vi "String-Matrix.vi"(10 "String":string) -> (0 "error out":errorcluster, 2 "String Out":string, 3 "T":T1=[[0.016284994521607307, 0.9998576764567041, 0.0044074691186384496, -12.095922523672678], [0.9998670931969393, -0.01628143110047913, -0.0008431744914288715, -1019.3924117975101], [-0.0007712945830650122, 0.004420614427981981, -0.999989931585686, 240.25900755427352], [0.0, 0.0, 0.0, 1.0]] format="%.3f")   [LabVIEW 2013]
uses:
  <vilib>/Analysis/Matrix/Datatypes/RealMatrix.ctl
  <vilib>/Analysis/Matrix/NI_Matrix.lvlib
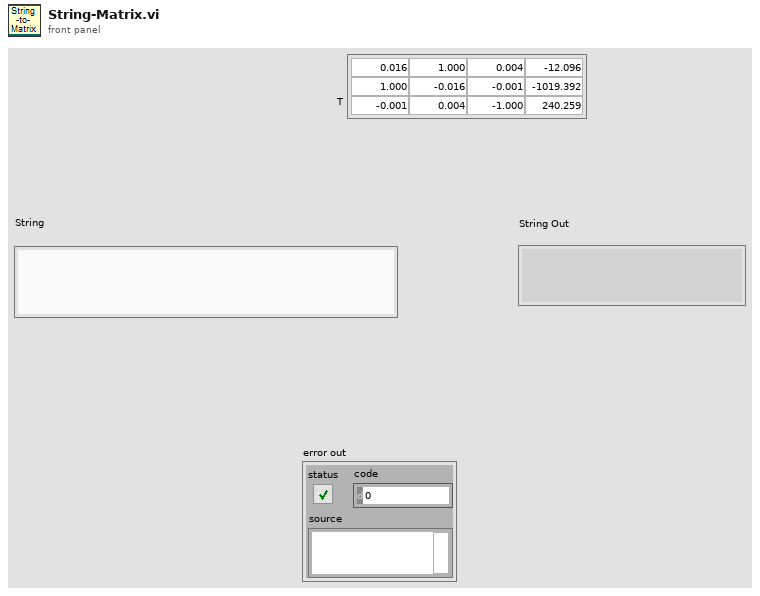
[diagram p1: front panel]
types:
  T1 = typedef "NI_Matrix.lvlib/RealMatrix.ctl" = dbl[][]
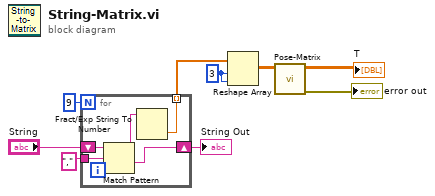
[diagram p0: block diagram]
diagram:
  w6 = 3 ("dimension size")
  n1 = for {
    N: 9 -> [_]
    shift-right: [w11] -> w1
    shift-left: "String" -> [w14]
    tunnel: [w12] -> w7 mode=indexing
    tunnel: "," ("regular expression") -> [w10]
    n2 = Match Pattern(string=w14, regular expression=w10) -> (before substring=w13:string, after substring=w11:string)  [unwired: 1 in, 2 out]
    n3 = Fract/Exp String To Number(string=w13) -> (number=w12:dbl)  [unwired: 3 in, 1 out]
  }
  "String Out" <- w1
  n4 = Reshape Array(w7, w6, w6) -> (w5:dbl[][])
  n5 = call "Pose-Matrix.vi"("pose"=w5) -> ("error out"=→"error out":errorcluster, "T"=→"T":T1)  [unwired: 9 in]
